vi "sendOutputData.vi"(8 "error in (no error)":errorcluster, 11 "Model in":refnum<class "Model.lvclass">) -> (0 "error out":errorcluster, 3 "Model out":refnum<class "Model.lvclass">)   [LabVIEW 2015, in "Model.lvclass"]
uses:
  Model.lvclass
  Typedefs/OutputData.ctl
  Model.lvclass/Model.ctl
  UserEvents/UserEvents.lvclass/UserEvents.ctl
  <userlib>/Common/ILC/ILC/ILC.lvclass/ILC.ctl
  <userlib>/Common/ILC/ILC/ILC.lvclass
  Typedefs/AITDTTypedefs.lvlib
  UserEvents/UserEvents.lvclass
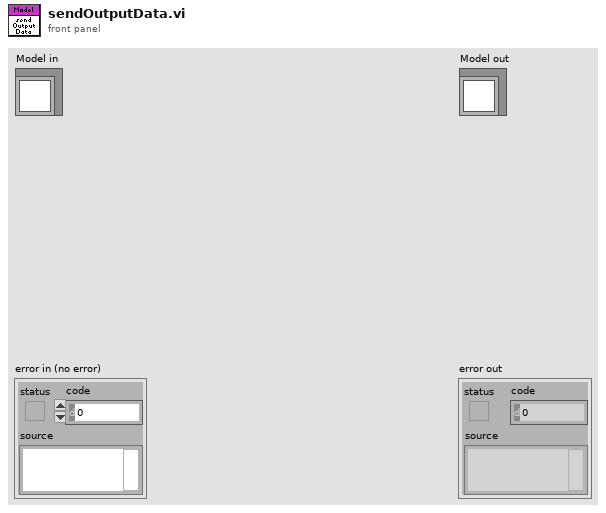
[diagram p1: front panel]
types:
  T1 = typedef "AITDTTypedefs.lvlib/OutputData.ctl" = cluster{"Step & Direction":i16}
  T2 = typedef "ILCCommon.lvlib/ILCTypedefs.lvlib/OutputData.ctl" = cluster{"Step & Direction":i16, "Blower RPM":u8, "PWM (SSR)":u8, "Ch1":u16, "Ch2":u16, "Ch3":u16, "Ch4":u16}
  T3 = typedef "AITDTTypedefs.lvlib/PubDataEvents.ctl" = cluster{"State":refnum<user-event>, "ErrorCode":refnum<user-event>, "OutputData":refnum<user-event>, "InputData":refnum<user-event>, "TestStatus":refnum<user-event>, "LogPath":refnum<user-event>, "TemperatureSetpointRequest":refnum<user-event>, "TemperatureSettling":refnum<user-event>, "WaitTimeStatus":refnum<user-event>}
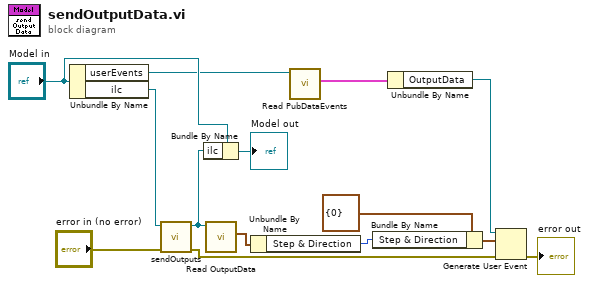
[diagram p0: block diagram]
diagram:
  n1 = Unbundle By Name("Model in") -> ("userEvents"=w3:refnum<class "UserEvents.lvclass">, "ilc"=w11:refnum<class "ILC.lvclass">)
  n2 = call <userlib>:"sendOutputs.vi"("error in (no error)"="error in (no error)", "ILC in"=w11) -> ("error out"=w2:errorcluster, "ILC out"=w9:refnum<class "ILC.lvclass">)  [unwired: 8 in]
  n3 = Bundle By Name(cluster="Model in", "ilc"=w9) -> (→"Model out":refnum<class "Model.lvclass">)
  n4 = call <userlib>:"Read OutputData.vi"("ILC in"=w9) -> ("OutputData"=w7:T2)  [unwired: 9 in, 1 out]
  n5 = Unbundle By Name(w7) -> ("Step & Direction"=w1:i16)
  n6 = call "Read PubDataEvents.vi"("UserEvents in"=w3) -> ("PubDataEvents"=w5:T3)  [unwired: 9 in, 1 out]
  n7 = Bundle By Name(cluster=T1 {"Step & Direction"=0} ("event data"), "Step & Direction"=w1) -> (w6:T1)
  n8 = Unbundle By Name(w5) -> ("OutputData"=w4:refnum<user-event>)
  n9 = Generate User Event(user event=w4, event data cluster=w6, error in=w2) -> (error out=→"error out":errorcluster)  [unwired: 1 in, 1 out]
